vi "A_times_x_fxp.vi"(9 "Az_mat in":fxp<+/-,32,5>[][](array[numeric]), 10 "x_k":fxp<+/-,32,5>[](array[numeric])=[0.0, 0.0, 0.0, 0.0, 0.0, 0.0, 0.0, 0.0, 0.0, 0.0, 0.0, 0.0, 0.0, 0.0, 0.0, 0.0, 0.0, 0.0, 0.0, 0.0, 0.0, 0.0, 0.0, 0.0, 0.0, 0.0, 0.0, 0.0, 0.0, 0.0, 0.0, 0.0, 0.0, 0.0, 0.0, 0.0, 0.0, 0.0, 0.0, 0.0, 0.0, 0.0, 0.0, 0.0, 0.0, 0.0, 0.0, 0.0, 0.0, 0.0]) -> (2 "A*x":fxp<+/-,64,12>[](array[numeric]), 3 "Az_vec out":fxp<+/-,32,5>[](array[numeric]))   [LabVIEW 2017]
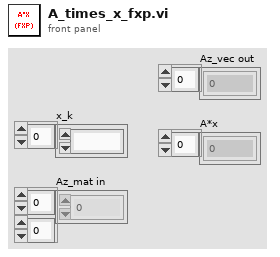
[diagram p1: front panel]
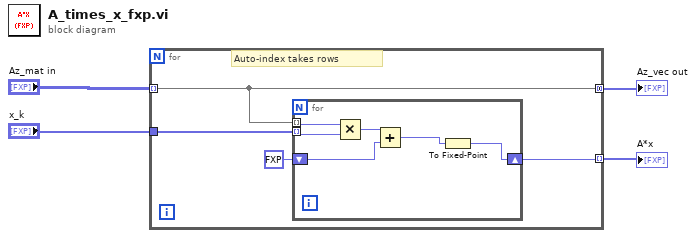
[diagram p0: block diagram]
diagram:
  n1 = for {
    tunnel: "Az_mat in" -> [w8] mode=indexing
    tunnel: [w8] -> w3 mode=concatenating
    tunnel: "x_k" -> [w7]
    tunnel: [w5] -> w4 mode=indexing
    # "Auto-index takes rows"
    n2 = for {
      tunnel: w8 -> [w14] mode=indexing
      tunnel: w7 -> [w13] mode=indexing
      shift-right: [w9] -> w5
      shift-left: fxp<+,1,1> 0.0 -> [w11]
      n3 = Multiply(x=w14, y=w13) -> (x*y=w12:fxp<+/-,64,10>)
      n4 = Add(x=w12, y=w11) -> (x+y=w10:fxp<+/-,64,13>)
      n5 = To Fixed-Point(number=w10) -> (fixed-point=w9:fxp<+/-,64,12>)  [unwired: 1 in]
    }
  }
  "A*x" <- w4
  "Az_vec out" <- w3
